vi "GOOP_VI_Provider_OnCommand.vi"(10 "Command Tag":string, 11 "objects":T1[](array[typedef])) -> ()   [LabVIEW 2020]
uses:
  <resource>/Framework/Providers/API/ItemRef.ctl
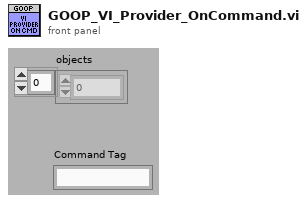
[diagram p1: front panel]
types:
  T1 = typedef "ItemRef.ctl" = u64
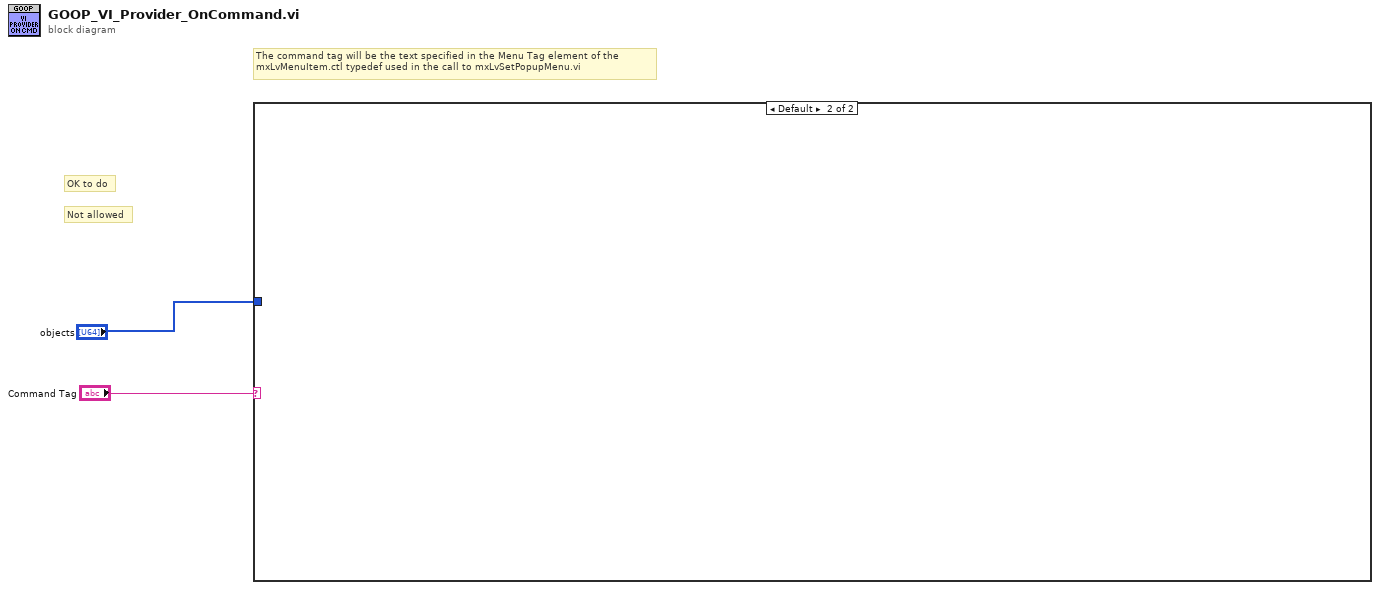
[diagram p0: block diagram]
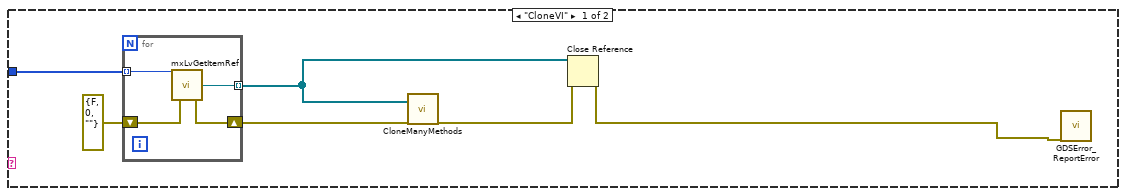
[diagram p2: hidden frame]
diagram:
  # "Not allowed"
  # "OK to do"
  # "The command tag will be the text specified in the Menu Tag element of the \nmxLvMenuItem.ctl typedef used in the call to mxLvSetPopupMenu.vi"
  n1 = case shown="Default" "Command Tag" {
    tunnel: "objects" -> [w7 _]
    frame "CloneVI" {
      n2 = for {
        tunnel: w7 -> [w12] mode=indexing
        tunnel: [w11] -> w4 mode=indexing
        shift-right: [w10] -> w6
        shift-left: errorcluster {"status"=FALSE, "code"=0, "source"=""} ("error out") -> [w9]
        n3 = call <resource>:"mxLvGetItemRef.vi"("Item"=w12, "error in"=w9) -> ("Item Refnum"=w11:refnum<vi>, "error out"=w10:errorcluster)  [unwired: 1 out]
      }
      n4 = call <resource>:"CloneManyMethods.vi"("VIRefs"=w4, "error in (no error)"=w6) -> ("error out"=w3:errorcluster)  [unwired: 16 in, 1 out]
      n5 = Close Reference(reference=w4, error in (no error)=w3) -> (error out=w8:errorcluster)
      n6 = call <resource>:"GDSError_ReportError.vi"("error in (no error)"=w8) -> ()  [unwired: 18 in, 1 out]
    }
    frame Default {
    }
  }
